vi "C3_Create.vi"(8 "error in (no error)":errorcluster, 11 "reference in":refnum<class "C3.lvclass">) -> (0 "error out":errorcluster, 3 "reference out":refnum<class "C3.lvclass">)   [LabVIEW 2012, in "C3.lvclass"]
uses:
  C3.lvclass
  B3_class/B3.lvclass
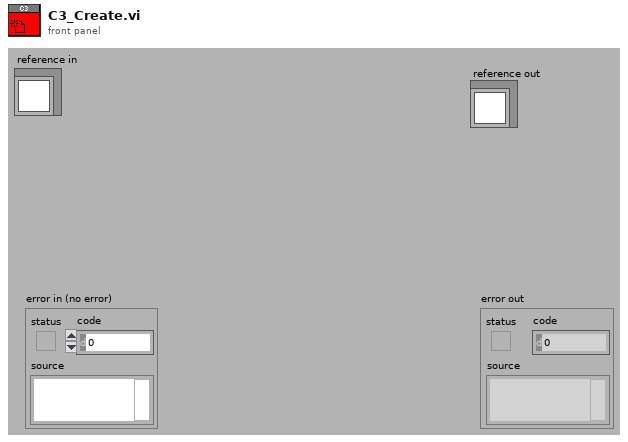
[diagram p1: front panel]
types:
  T1 = typedef "C3.lvclass/ObjectAttributes.ctl" = cluster{"Base class":T2}
  T2 = typedef "B3.lvclass/ObjectAttributes.ctl" = cluster{"Base class":T3}
  T3 = typedef "A3.lvclass/ObjectAttributes.ctl" = cluster{"Attribute1":dbl}
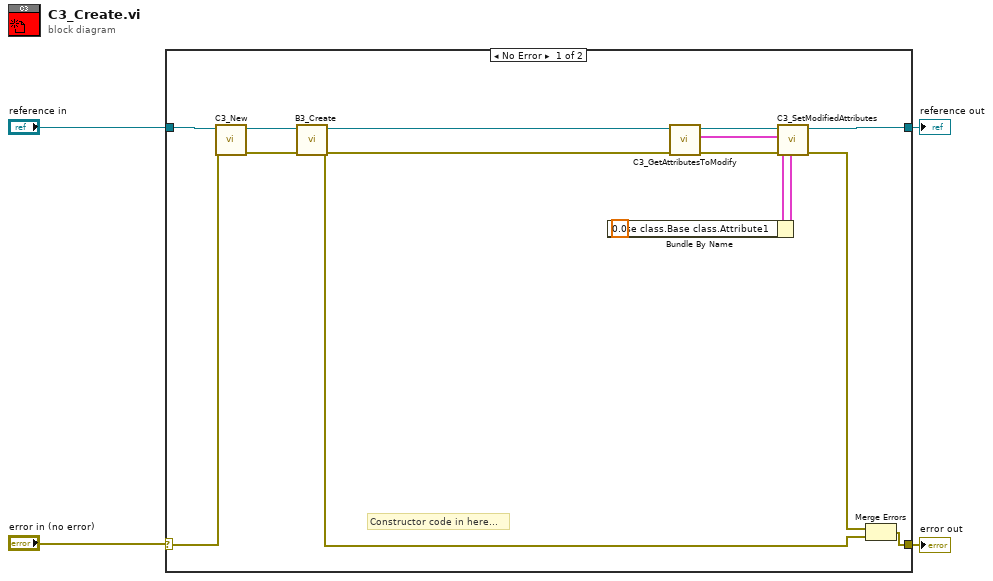
[diagram p0: block diagram]
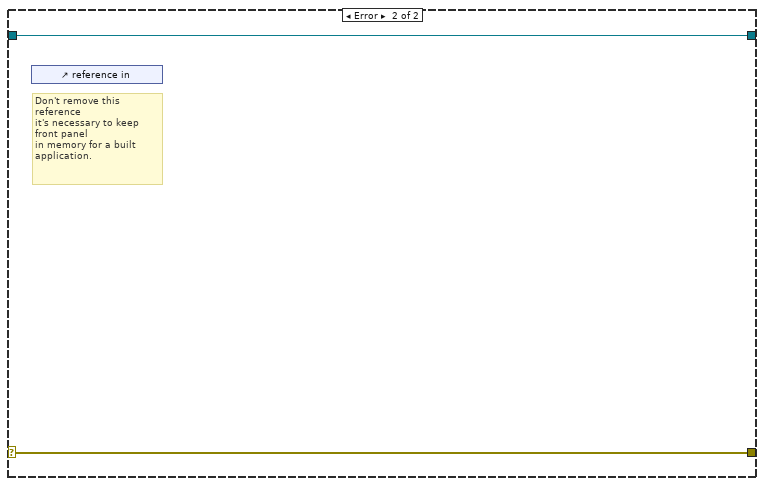
[diagram p2: hidden frame]
diagram:
  n1 = case shown="No Error" "error in (no error)" {
    selector: "error in (no error)" -> [w16 w20]
    tunnel: [w9 w20] -> w3
    tunnel: [w14 w19] -> w2
    tunnel: "reference in" -> [w6 w19]
    frame No Error {
      # "Constructor code in here..."
      n2 = call "C3_New.vi"("error in (no error)"=w16, "reference in"=w6) -> ("error out"=w15:errorcluster, "reference out"=w11:refnum<class "C3.lvclass">)  [unwired: 6 in, 2 out]
      n3 = call "B3_Create.vi"("error in (no error)"=w15, "reference in"=w11) -> ("error out"=w7:errorcluster, "reference out"=w10:refnum<class "C3.lvclass">)  [unwired: 8 in]
      n4 = call "C3_GetAttributesToModify.vi"("error in (no error)"=w7, "reference in"=w10) -> ("error out"=w17:errorcluster, "Attributes"=w13:T1, "reference out"=w18:refnum<class "C3.lvclass">)  [unwired: 6 in, 1 out]
      n5 = Bundle By Name(cluster=w13, "Base class.Base class.Attribute1"=0.0 ("Base class.Attribute1")) -> (w12:T1)
      n6 = call "C3_SetModifiedAttributes.vi"("error in (no error)"=w17, "Attributes"=w12, "reference in"=w18) -> ("error out"=w8:errorcluster, "reference out"=w14:refnum<class "C3.lvclass">)  [unwired: 7 in]
      n7 = Merge Errors(w8, w7) -> (w9:errorcluster)
    }
    frame Error {
      # "Don't remove this reference\nit's necessary to keep front panel\nin memory for a built application."
      n8 = control-ref of="reference in"() -> ()  [unwired: 1 out]
    }
  }
  "error out" <- w3
  "reference out" <- w2
